vi "sv_Prepare Acquired Waveforms for Parsing_Copy.vi"(4 "append virtual reference":bool, 6 "propagation delay":T1, 7 "restart (F)":bool, 8 "error in":errorcluster, 9 "SV Signal":refnum<class "SV Signal.lvclass">, 11 "acquired channel waveforms":waveform(dbl)[](array[waveform])) -> (0 "error out":errorcluster, 3 "aligned channel waveforms":waveform(dbl)[](array[waveform]), 5 "alignment reference detected":bool)   [LabVIEW 2021, in "Audio ADC Shared.lvlib"]
doc: "Align signals and optionally append virtual reference prior to writing data to SV Buffer and parsing for measurement samples."
uses:
  Audio ADC Shared.lvlib
  <vilib>/addons/_NISVFA/_Generation/Signal Generation/SV Signal/SV Signal.lvclass
  <vilib>/addons/_NISVFA/_Generation/Signal Generation/SV Signal/SV Signal.lvclass/SV Signal.ctl
  <vilib>/addons/_NISVFA/_Generation/Signal Generation/SV Signal/Read Synchronization Pulse Waveform.vi
  Program Files/National Instruments/LabVIEW 2021/examples/Sound and Vibration/Audio Measurements/subVIs/sv_Measure Delay for Active and Idle Channels.vi
  <vilib>/addons/_NISVFA/_Generation/Signal Generation/SV Signal/Read Leading Synchronization Pulse Enable.vi
  <vilib>/addons/_NISVFA/_Generation/Signal Generation/SV Signal/Read Trailing Synchronization Pulse Enable.vi
  <vilib>/addons/_NISVFA/_Generation/Signal Generation/SV Signal/Write Leading Synchronization Pulse Enable.vi
  <vilib>/addons/_NISVFA/_Shared subVIs/Common/svc_Check for Waveform Parameter Continuity (no state).vi
  <vilib>/addons/_NISVFA/_Shared subVIs/Common/sv_Get NI Property Name String.vi
  <vilib>/addons/Sound and Vibration/svt_Calibration/SV Measure Delay and Polarity and Coherence (Nx1).vi
  Program Files/National Instruments/LabVIEW 2021/examples/Sound and Vibration/Audio Measurements/subVIs/sv_Assign Delay to Idle Channels.vi
  <vilib>/addons/_NISVFA/_Shared subVIs/Common/svc_Get SV Channel Info.vi
  <vilib>/addons/Sound and Vibration/svt_Calibration/SV Measure Delay and Polarity and Coherence.vi
  <vilib>/addons/_NISVFA/_Shared subVIs/Common/svc_Unit Label to Engineering Units.vi
  <vilib>/addons/_NISVFA/_Shared subVIs/Common/svc_Engineering Units to Unit Label.vi
  <vilib>/Analysis/_algsub.llb/Vector Norm.vi
  <vilib>/Analysis/_algsub.llb/Real Vector Norm.vi
  <vilib>/addons/_NISVFA/_Shared subVIs/Common/SV Get Data Subset.vi
  <vilib>/addons/_NISVFA/_Shared subVIs/Common/svc_Get Array Subset (Index).vi
  <vilib>/addons/_NISVFA/_Shared subVIs/Common/svc_Coerce Index and Length.vi
  <vilib>/addons/_NISVFA/_Shared subVIs/Common/svc_Conditional Merge Error.vi
  <vilib>/addons/_NISVFA/_Generation/Signal Generation/SV Signal/Read System Timing Model.vi
  <vilib>/addons/_NISVFA/_Generation/Signal Generation/SV Signal/Write System Timing Model.vi
  <vilib>/addons/_NISVFA/_Shared subVIs/Data Objects/Waveforms (DBL)/Write to Buffer.vi
  <vilib>/addons/_NISVFA/_Shared subVIs/Data Objects/Waveforms (DBL)/Read from Buffer.vi
  <vilib>/addons/_NISVFA/_Shared subVIs/Data Objects/Waveforms (DBL)/SV Read Newest Data.vi
  <vilib>/measure/maresamp.llb/Resample Waveforms (single shot).vi
  <vilib>/measure/maresamp.llb/Resample Waveform (single shot).vi
  <vilib>/addons/_NISVFA/_Shared subVIs/Common/svc_Check dt for Equal Sample Rates.vi
  <vilib>/Waveform/TSOps.llb/Timestamp Subtract.vi
  <vilib>/Analysis/2dsp.llb/CrossCorrelation.vi
  <vilib>/Analysis/2dsp.llb/1D Cross Correlation (DBL).vi
  <vilib>/addons/_NISVFA/_Shared subVIs/Common/svc_Fit Quadratic to Max Three Points in Array.vi
  <vilib>/Utility/error.llb/Error Cluster From Error Code.vi
  <vilib>/addons/_NISVFA/_Shared subVIs/Common/svc_Caller VI Returned in Error Source.vi
  <vilib>/addons/_NISVFA/_Shared subVIs/Common/SV Remove Delays (1,N) from Waveforms (N Ch) (DBL).vi
  <vilib>/addons/_NISVFA/_Generation/Signal Generation/SV Signal/Read Sample Rate.vi
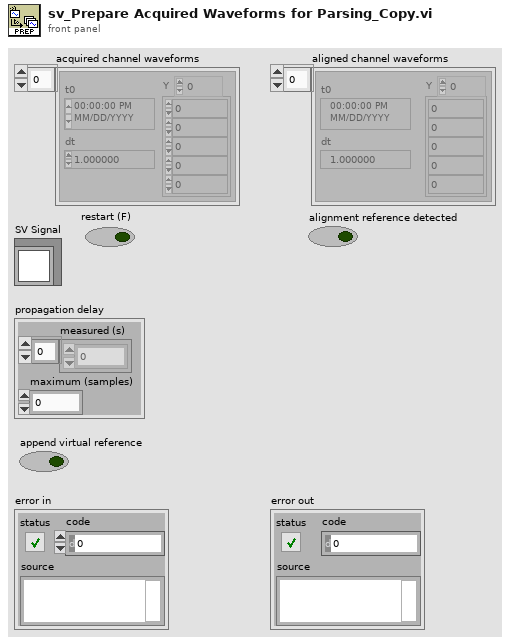
[diagram p1: front panel]
types:
  T1 = cluster{"measured (s)":dbl[], "maximum (samples)":i32}
  T2 = cluster{"dt equal":bool, "array length equal":bool, "number channels change":bool}
  T3 = cluster{"dt":bool, "t0 continuity":bool, "array length":bool, "channel info":bool, "name":bool}
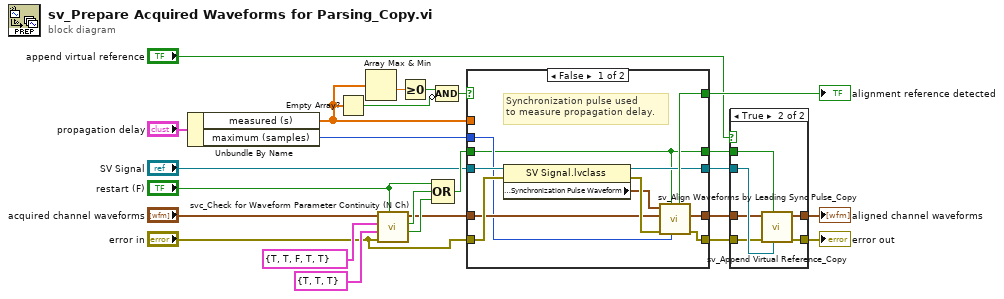
[diagram p0: block diagram]
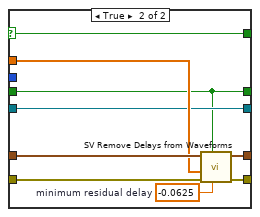
[diagram p3: hidden frame]
diagram:
  n1 = Unbundle By Name("propagation delay") -> ("measured (s)"=w25:dbl[], "maximum (samples)"=w2:i32)
  n2 = Empty Array?(array=w25) -> (empty?=w3:bool)
  n3 = Array Max & Min(array=w25) -> (min value=w22:dbl)  [unwired: 3 out]
  n4 = call <vilib>:"svc_Check for Waveform Parameter Continuity (N Ch).vi"("restart averaging (F)"="restart (F)", "error in"="error in", "checks for multichannel parameters"=T2 {"dt equal"=TRUE, "array length equal"=TRUE, "number channels change"=TRUE}, "checks for channel parameter change"=T3 {"dt"=TRUE, "t0 continuity"=TRUE, "array length"=FALSE, "channel info"=TRUE, "name"=TRUE}, "scaled signal(s)"="acquired channel waveforms") -> ("multichannel parameter changed"=w17:bool, "waveform parameter changed"=w18:bool, "dup scaled signal(s)"=w8:waveform(dbl)[])  [unwired: 4 out]
  n5 = Greater Or Equal To 0?(x=w22) -> (x >= 0?=w23:bool)
  n6 = Compound Arithmetic op=OR("restart (F)", w18, w17) -> (w19:bool)
  n7 = Compound Arithmetic op=AND(w23, invert w3) -> (w24:bool)
  n8 = case shown="False" w24 {
    selector: w24 -> [_ w41]
    tunnel: "error in" -> [w35 w43]
    tunnel: w8 -> [w34 w45]
    tunnel: "SV Signal" -> [w32 w39]
    tunnel: [w31 w42] -> w11
    tunnel: [w30 w44] -> w12
    tunnel: w25 -> [_ w40]
    tunnel: w2 -> [w29 _]
    tunnel: w19 -> [w26 w38]
    tunnel: [w28 w41] -> w21
    tunnel: [w27 w39] -> w7
    tunnel: [w26 w38] -> w6
    frame False {
      # "Synchronization pulse used \nto measure propagation delay."
      n9 = property on="Property Node" class="SV Signal.lvclass"(reference=w32, error in=w35) -> (reference out=w27:refnum<class "SV Signal.lvclass">, error out=w36:errorcluster, "Signal Properties:Synchronization Pulses:Synchronization Pulse Waveform"=w33:waveform(dbl))
      n10 = call "sv_Align Waveforms by Leading Sync Pulse_Copy.vi"("maximum delay"=w29, "reset"=w26, "error in (no error)"=w36, "response signals"=w34, "alignment reference signal"=w33) -> ("error out"=w31:errorcluster, "aligned signals"=w30:waveform(dbl)[], "alignment reference detected"=w28:bool)  [unwired: 2 in, 2 out]
    }
    frame True {
      w37 = -0.0625  # minimum residual delay
      n11 = call-poly <vilib>:"SV Remove Delays from Waveforms.vi"("minimum residual delay"=w37, "reset"=w38, "error in (no error)"=w43, "path-dependent analog delays [s]"=w40, "scaled signals"=w45) -> ("error out"=w42:errorcluster, "aligned signals"=w44:waveform(dbl)[])  [unwired: 3 in, 2 out]
    }
  }
  "alignment reference detected" <- w21
  n12 = case shown="True" "append virtual reference" {
    tunnel: [w47 w53] -> w5
    tunnel: w7 -> [_ w52]
    tunnel: [w46 w51] -> w4
    tunnel: w12 -> [w47 w50]
    tunnel: w11 -> [w46 w49]
    tunnel: w6 -> [_ w48]
    frame False {
    }
    frame True {
      n13 = call "sv_Append Virtual Reference_Copy.vi"("SV Signal in"=w52, "reset"=w48, "error in (no error)"=w49, "acquired waveforms"=w50) -> ("error out"=w51:errorcluster, "acquired waveforms with virtual reference"=w53:waveform(dbl)[])  [unwired: 6 in]
    }
  }
  "aligned channel waveforms" <- w5
  "error out" <- w4
